vi "Execute Write Request.vi"(9 "IWritePolicy in":refnum<class "IWriteStrategy.lvclass">, 10 "Connection Writer":refnum<class "ProtectedConnectionWriter.lvclass">, 11 "WriteRequest in":refnum<class "WriteRequest.lvclass">) -> (0 "error out":errorcluster)   [LabVIEW 2020, in "MessagingInterfaces.lvlib" / "WriteRequest.lvclass"]
uses:
  <vilib>/gpm_packages/@cs/Network-interface/Source/MessagingInterfaces/WriteRequest/WriteRequest.lvclass
  <vilib>/gpm_packages/@cs/Network-interface/Source/MessagingInterfaces/IWriteStrategy/IWriteStrategy.lvclass
  <vilib>/gpm_packages/@cs/Network-interface/Source/ProtectedConnectionWriter/ProtectedConnectionWriter.lvclass
  <vilib>/gpm_packages/@cs/Network-interface/Source/MessagingInterfaces/WriteRequest/WriteRequest.lvclass/WriteRequest.ctl
  <vilib>/gpm_packages/@cs/Network-interface/Source/MessagingInterfaces/IWriteExecutionCallback/IWriteExecutionCallback.lvclass
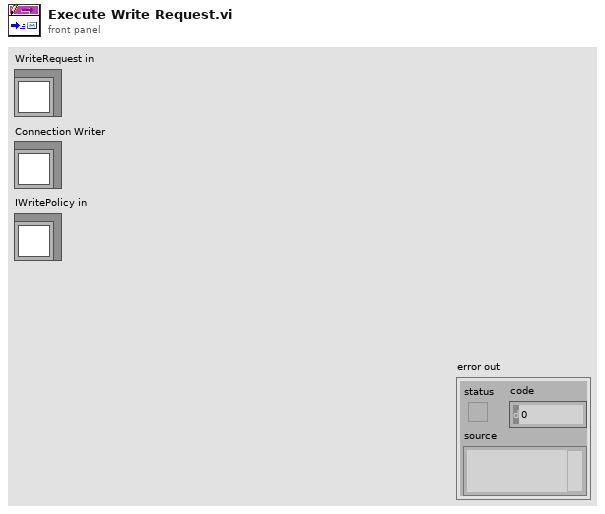
[diagram p1: front panel]
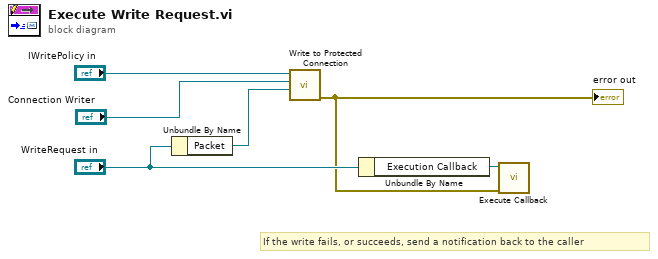
[diagram p0: block diagram]
diagram:
  # "If the write fails, or succeeds, send a notification back to the caller"
  n1 = Unbundle By Name("WriteRequest in") -> ("Packet"=w4:refnum<class "IPacket.lvclass">)
  n2 = call-dynamic "Write to Protected Connection.vi"("Packet"=w4, "Connection Writer"="Connection Writer", "IWriteStrategy in"="IWritePolicy in") -> ("error out"=w1:errorcluster)  [unwired: 8 in]
  "error out" <- w1
  n3 = Unbundle By Name("WriteRequest in") -> ("Execution Callback"=w2:refnum<class "IWriteExecutionCallback.lvclass">)
  n4 = call-dynamic "Execute Callback.vi"("Write Status"=w1, "IWriteExecutionPolicy in"=w2) -> ()  [unwired: 10 in]
